vi "lightsMotorsFans.vi"() -> ()   [LabVIEW 2019]
panel:
  in  "Motor 1":i32 min=0 max=99999 format="%05.0f"
  in  "Light 1":i32 min=0 max=1 format="%01.0f"
  in  "Light 2":i32 min=0 max=1 format="%01.0f"
  in  "Light 3":i32 min=0 max=1 format="%01.0f"
  in  "Fans":i32 min=0 max=1 format="%01.0f"
  in  "Motor 10":i32 min=0 max=99999 format="%05.0f"
  in  "Motor 9":i32 min=0 max=99999 format="%05.0f"
  in  "Motor 8":i32 min=0 max=99999 format="%05.0f"
  in  "Motor 7":i32 min=0 max=99999 format="%05.0f"
  in  "Motor 6":i32 min=0 max=99999 format="%05.0f"
  in  "Motor 5":i32 min=0 max=99999 format="%05.0f"
  in  "Motor 4":i32 min=0 max=99999 format="%05.0f"
  in  "Motor 3":i32 min=0 max=99999 format="%05.0f"
  in  "Motor 2":i32 min=0 max=99999 format="%05.0f"
  in  "VISA- Arduino Mega":refnum<visa-resource-name>
  in  "stop":bool
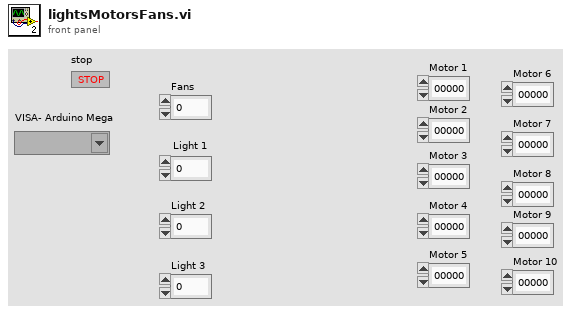
[diagram p1: front panel]
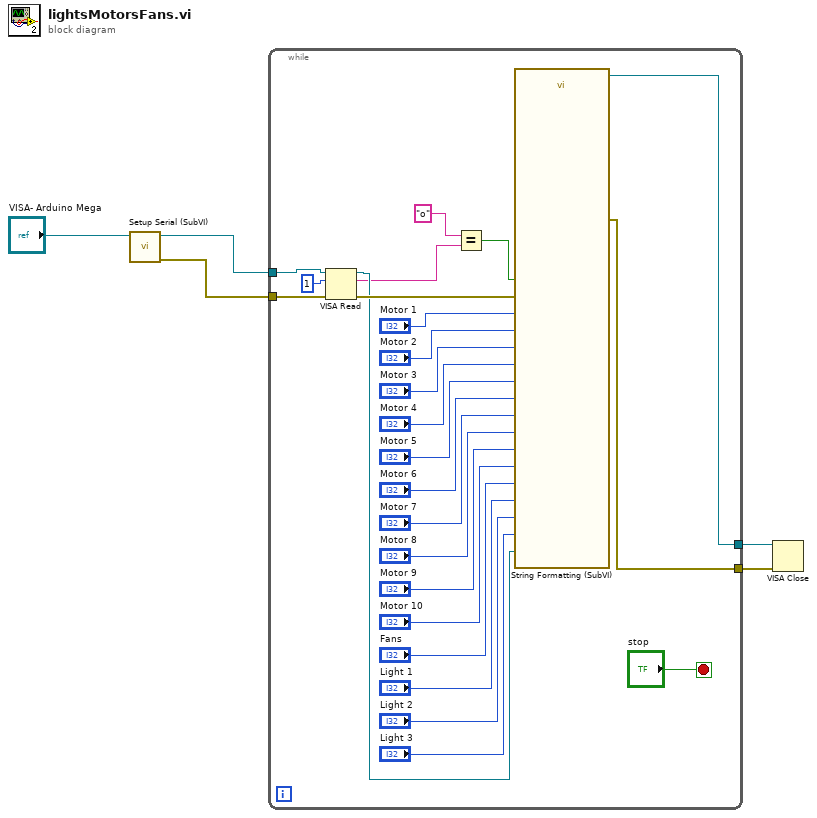
[diagram p0: block diagram]
diagram:
  n1 = call "Setup Serial (SubVI).vi"("VISA Refnum in"="VISA- Arduino Mega") -> ("error out"=w1:errorcluster, "VISA Refnum out"=w2:refnum<visa-resource-name>)  [unwired: 9 in]
  n2 = while {
    tunnel: w1 -> [w23]
    tunnel: w2 -> [w22]
    tunnel: [w24] -> w4
    tunnel: [w25] -> w3
    stop <- "stop" stop-if-true
    n3 = VISA Read(VISA resource name=w22, byte count=u32 1, error in (no error)=w23) -> (VISA resource name out=w27:refnum<visa-resource-name>, read buffer=w8:string, error out=w28:errorcluster)  [unwired: 1 out]
    n4 = Equal?(x="o" ("y"), y=w8) -> (x = y?=w29:bool)
    n5 = call "String Formatting (SubVI).vi"("VISA Refnum in"=w27, "Motor 6"="Motor 6", "Light 1"="Light 1", "Motor 7"="Motor 7", "Light 2"="Light 2", "Motor 8"="Motor 8", "Motor 9"="Motor 9", "error in (no error)"=w28, "Motor 5"="Motor 5", "Motor 10"="Motor 10", "Motor 4"="Motor 4", "Fans"="Fans", "Motor 3"="Motor 3", "Light 3"="Light 3", "Motor 2"="Motor 2", "Motor 1"="Motor 1", "Boolean"=w29) -> ("VISA Refnum out"=w25:refnum<visa-resource-name>, "error out"=w24:errorcluster)  [unwired: 8 in, 1 out]
  }
  n6 = VISA Close(VISA resource name=w3, error in (no error)=w4) -> ()  [unwired: 1 out]
